vi "PulseGeneratorSetParameters.vi"(0 "stimulus specifier":T3, 2 "stimulus parameters":T1) -> (3 "stimulus specifier 2":T3, 4 "stimulus information":T2, 5 "stimulus parameters":T1, 6 "error IO":errorcluster)   [LabVIEW 2014]
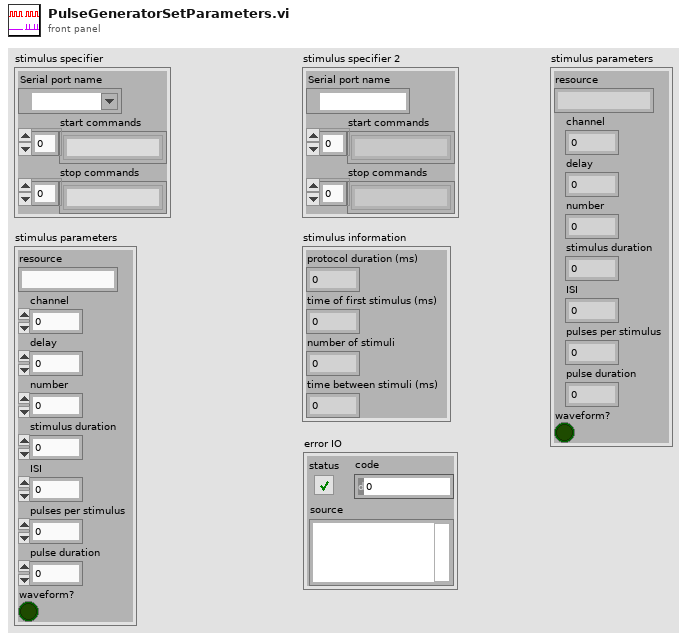
[diagram p1: front panel]
types:
  T1 = cluster{"resource":string, "channel":u16, "delay":dbl, "number":i32, "stimulus duration":dbl, "ISI":dbl, "pulses per stimulus":u16, "pulse duration":dbl, "waveform?":bool}
  T2 = cluster{"protocol duration (ms)":i64, "time of first stimulus (ms)":i64, "number of stimuli":u16, "time between stimuli (ms)":i64}
  T3 = cluster{"Serial port name":refnum<visa-resource-name>, "start commands":string[], "stop commands":string[]}
  T4 = cluster{dbl, "Number\nof stimuli":u16, dbl, dbl, "Pulses per\nstimulus":u16, dbl}
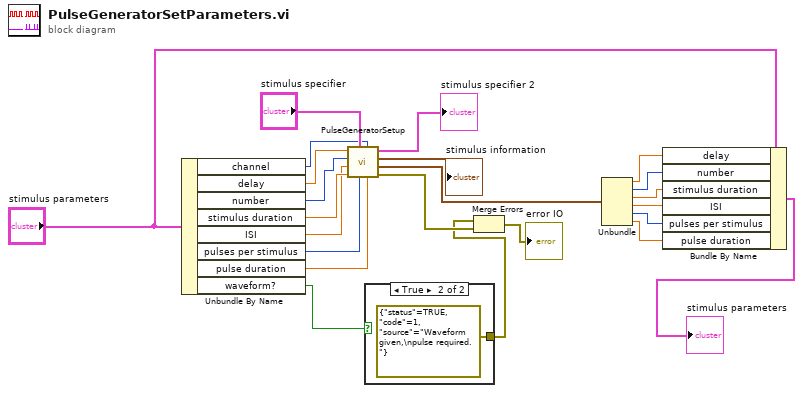
[diagram p0: block diagram]
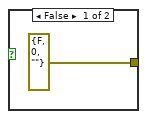
[diagram p2: hidden frame]
diagram:
  n1 = Unbundle By Name("stimulus parameters") -> ("channel"=w22:u16, "delay"=w16:dbl, "number"=w17:i32, "stimulus duration"=w19:dbl, "ISI"=w18:dbl, "pulses per stimulus"=w20:u16, "pulse duration"=w21:dbl, "waveform?"=w13:bool)
  n2 = call "PulseGeneratorSetup.vi"("Pulse duration (s)\nif more than one pulse"=w21, "Channel"=w22, "Pulses per\nstimulus"=w20, "stimulus specifier"="stimulus specifier", "Stimulus\nduration (s)"=w19, "Time between stimuli,\nstart-to-start (s)"=w18, "Number\nof stimuli"=w17, "Initial delay (s)"=w16) -> ("error IO"=w12:errorcluster, "stimulus parameters"=w9:T4, "stimulus information"=→"stimulus information":T2, "stimulus specifier"=→"stimulus specifier 2":T3)
  n3 = case shown="True" w13 {
    tunnel: [errorcluster {"status"=FALSE, "code"=0, "source"=""} ("error constant") errorcluster {"status"=TRUE, "code"=1, "source"="Waveform given,\npulse required."} ("error constant")] -> w11
    frame False {
    }
    frame True {
    }
  }
  n4 = Merge Errors(w11, w12) -> (→"error IO":errorcluster)
  n5 = Unbundle(w9) -> (w7:dbl, "Number\nof stimuli"=w6:u16, w5:dbl, w2:dbl, "Pulses per\nstimulus"=w3:u16, w4:dbl)
  n6 = Bundle By Name(cluster="stimulus parameters", "delay"=w7, "number"=w6, "stimulus duration"=w5, "ISI"=w2, "pulses per stimulus"=w3, "pulse duration"=w4) -> (→"stimulus parameters":T1)
